vi "main.vi"() -> ()   [LabVIEW 2018]
uses:
  ctl/matrix.ctl
  <vilib>/Utility/miscctls.llb/LVRectTypeDef.ctl
  <vilib>/Utility/error.llb/DialogType.ctl
panel:
  in  "选择模式":enum16{"模式一", "模式二"}(ring)
  in  "状态刷新":bool=TRUE
  out "系统时间":timestamp format="%<%.0X\n%x>T"
  in  "setting":T1
  in  "记录数据":i32=1 min=1 step=1
  out "系统状态":string
  out "运行中":bool
  in  "初始化":T1
  in  "停止":T1
  in  "开始测试":T1
  in  "停止变量":bool=TRUE
  out "第二行":T2
  out "第一行":T2
  # "气罐压力信号数据采集系统"
  # "轮"
  # "X1\n丨"
  # "X5\n丨"
  # "X10\n 丨"
  # "X15\n 丨"
  # "X20\n 丨"
  # "X25\n 丨"
  # "X30\n 丨"
  # "X35\n 丨"
  # "X40\n 丨"
  # "X45\n 丨"
  # "X50\n 丨"
  # "X55\n 丨"
  # "X60\n 丨"
  # "X64\n 丨"
  # "Y1一"
  # "Y2一"
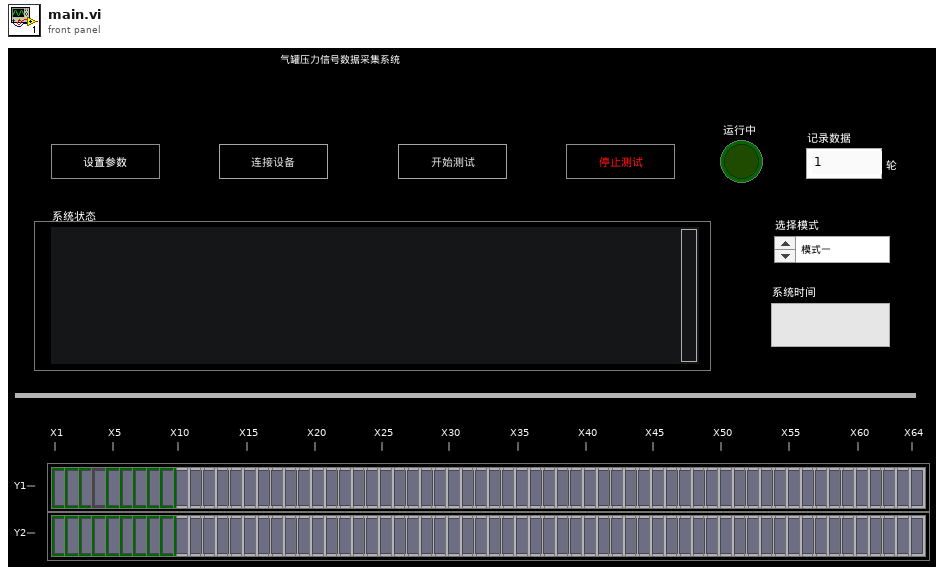
[diagram p1: front panel]
types:
  T1 = typedef "空白按钮.ctl" = bool
  T2 = typedef "matrix.ctl" = cluster{"布尔":bool, "布尔 2":bool, "布尔 3":bool, "布尔 4":bool, "布尔 5":bool, "布尔 6":bool, "布尔 7":bool, "布尔 8":bool, "布尔 9":bool, "布尔 10":bool, "布尔 11":bool, "布尔 12":bool, "布尔 13":bool, "布尔 14":bool, "布尔 15":bool, "布尔 16":bool, "布尔 17":bool, "布尔 18":bool, "布尔 19":bool, "布尔 20":bool, "布尔 21":bool, "布尔 22":bool, "布尔 23":bool, "布尔 24":bool, "布尔 25":bool, "布尔 26":bool, "布尔 27":bool, "布尔 28":bool, "布尔 29":bool, "布尔 30":bool, "布尔 31":bool, "布尔 32":bool, "布尔 33":bool, "布尔 34":bool, "布尔 35":bool, "布尔 36":bool, "布尔 37":bool, "布尔 38":bool, "布尔 39":bool, "布尔 40":bool, "布尔 41":bool, "布尔 42":bool, "布尔 43":bool, "布尔 44":bool, "布尔 45":bool, "布尔 46":bool, "布尔 47":bool, "布尔 48":bool, "布尔 49":bool, "布尔 50":bool, "布尔 51":bool, "布尔 52":bool, "布尔 53":bool, "布尔 54":bool, "布尔 55":bool, "布尔 56":bool, "布尔 57":bool, "布尔 58":bool, "布尔 59":bool, "布尔 60":bool, "布尔 61":bool, "布尔 62":bool, "布尔 63":bool, "布尔 64":bool}
  T3 = enum16{"错误", "关闭", "系统停止", "系统运行", "系统空闲", "初始化完成", "保存参数", "手动连接", "自动连接", "初始化"}
  T4 = enum32{"Invalid", "Standard", "Closed", "Hidden", "Minimized", "Maximized"}
  T5 = enum8{"Enabled", "Disabled", "Disabled and Grayed Out"}
  T6 = typedef "DialogType.ctl" = u16
  T7 = cluster{"矩阵卡设置":cluster{"BUS":u32, "slot":u32}, "模式一设置":cluster{"M1-drive-start":u32, "M1-drive-num":u32, "M1-receive-start":u32, "M1-receive-num":u32, "M1-start-delay":u32, "M1-receive-delay":u32}, "模式二设置":cluster{"M2-drive-start":u32, "M2-receive-start":u32, "M2-receive-num":u32, "M2-start-delay":u32, "M2-receive-delay":u32}, "采集设置":cluster{"Resource Name":refnum<k15>, "Input Impedance":u32, "采集通道":i32, "Trigger Level (V)":dbl, "Coupling":u16, "Trigger Slope":i32, "Min Record Length":i32, "Min. Sample Rate":dbl, "Vertical Range (V)":dbl, "触发通道":i32}}
  T8 = typedef "LVRectTypeDef.ctl" = cluster{"Left":i16, "Top":i16, "Right":i16, "Bottom":i16}
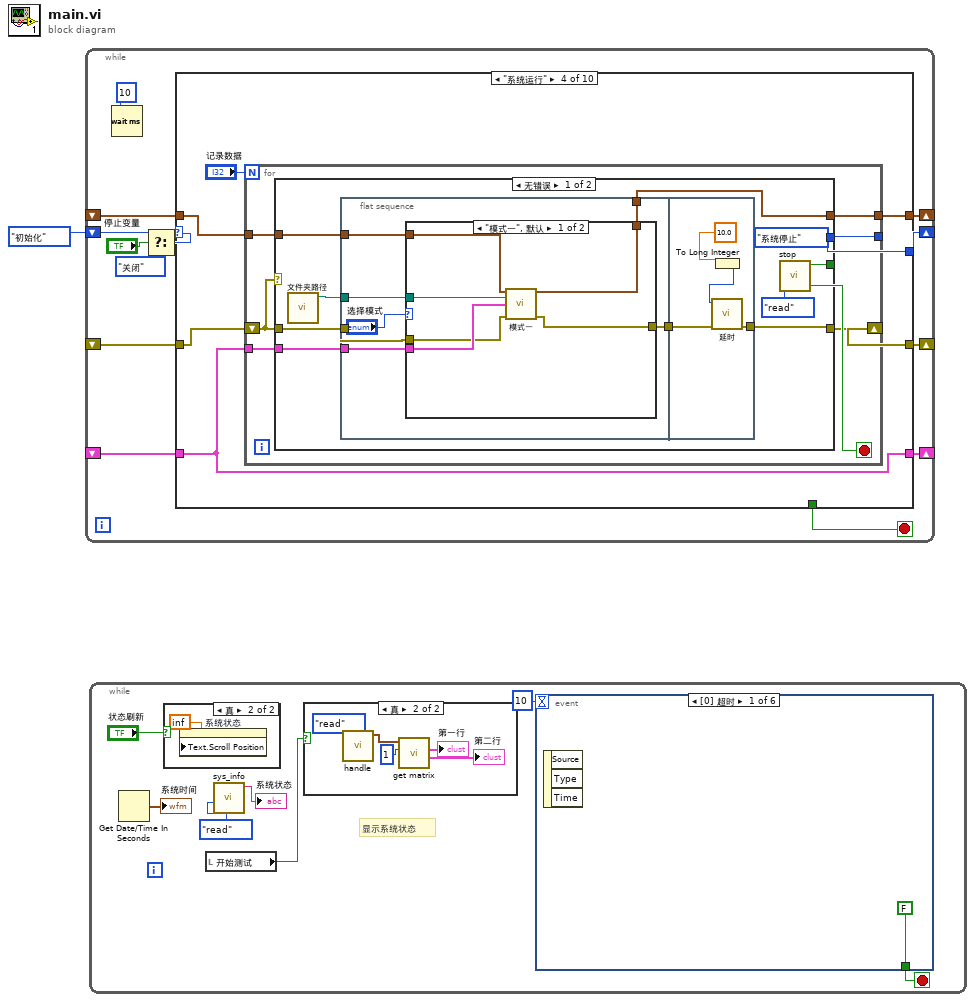
[diagram p0: block diagram]
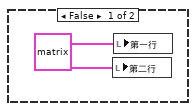
[diagram p2: hidden frame]
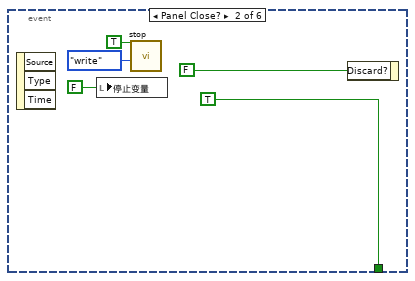
[diagram p4: hidden frame]
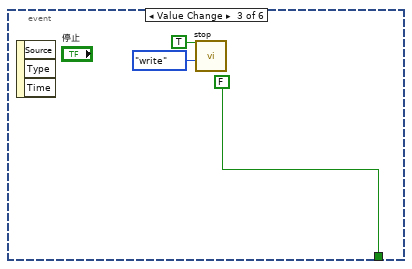
[diagram p5: hidden frame]
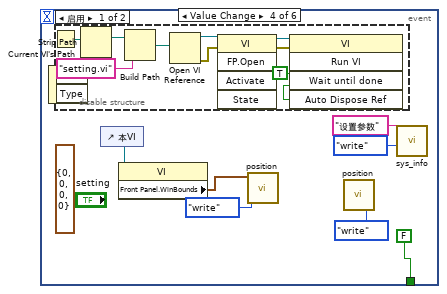
[diagram p6: hidden frame]
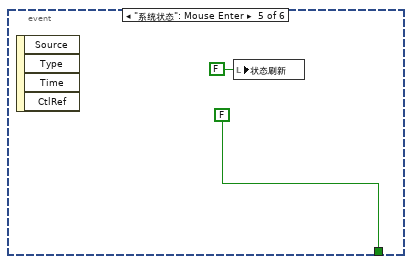
[diagram p8: hidden frame]
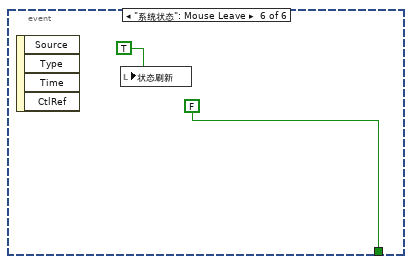
[diagram p9: hidden frame]
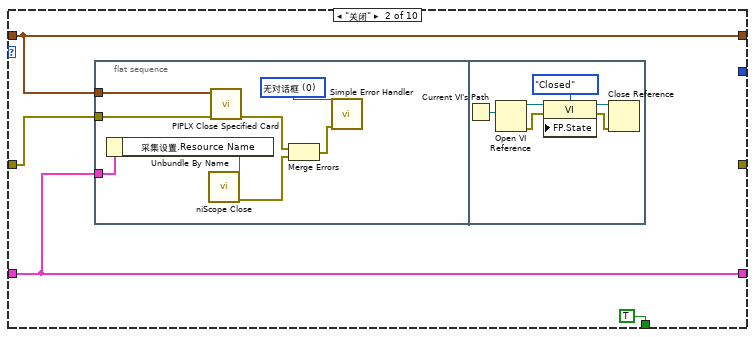
[diagram p11: hidden frame]
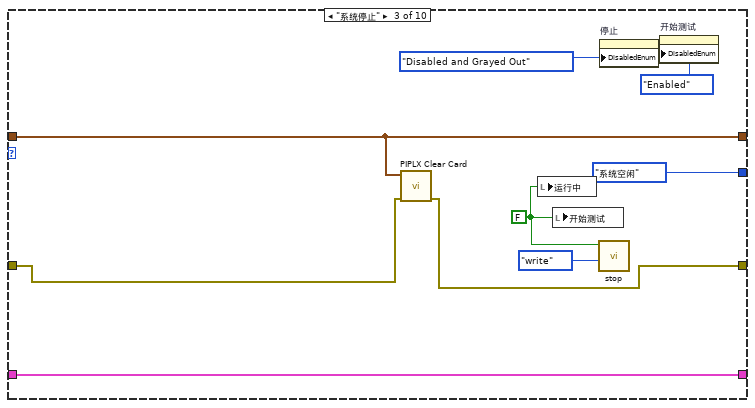
[diagram p12: hidden frame]
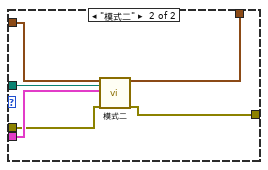
[diagram p13: hidden frame]
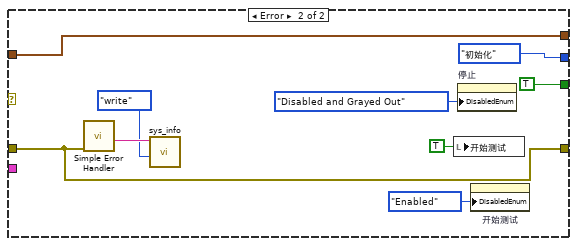
[diagram p14: hidden frame]
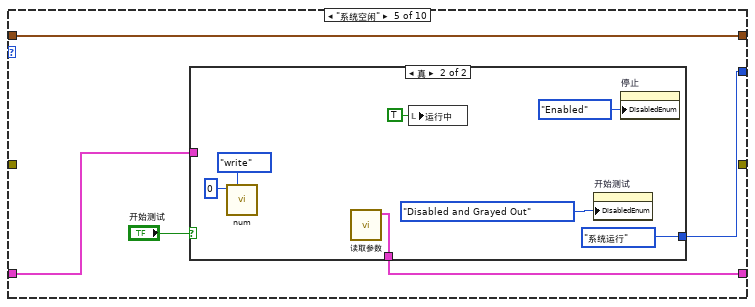
[diagram p15: hidden frame]
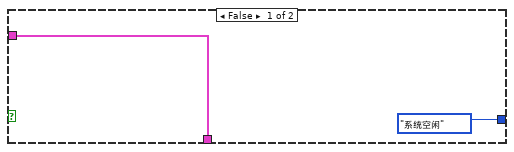
[diagram p16: hidden frame]
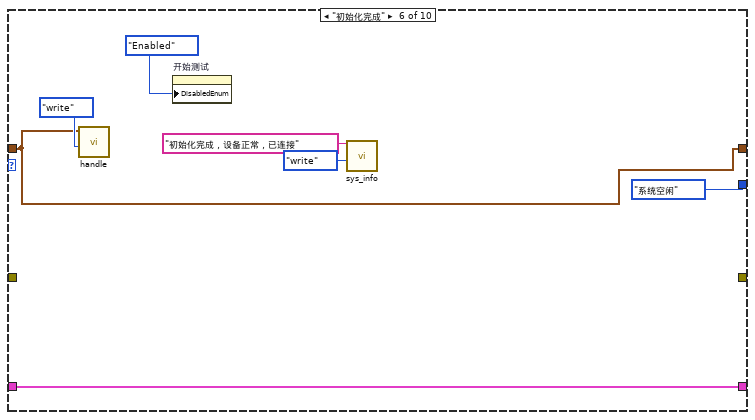
[diagram p17: hidden frame]
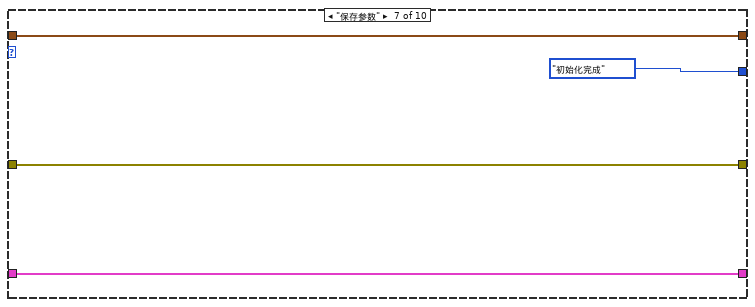
[diagram p18: hidden frame]
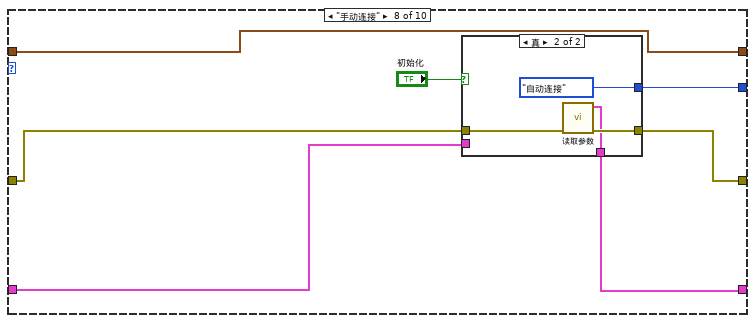
[diagram p19: hidden frame]
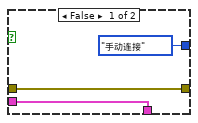
[diagram p20: hidden frame]
diagram:
  n1 = while {
    shift-right: [w14] -> _
    shift-left: T3."初始化" ("流程") -> [w12]
    shift-right: [w8] -> _
    shift-left: _ -> [w7]
    shift-right: [w5] -> _
    shift-left: _ -> [w4]
    shift-right: [w3] -> _
    shift-left: _ -> [w2]
    stop <- w6 stop-if-true
    n2 = Wait (ms)(milliseconds to wait=u32 10 ("等待时间（毫秒）")) -> ()  [unwired: 1 out]
    n3 = Select(t=w12, s="停止变量", f=T3."关闭") -> (s? t:f=w11:T3)
    n4 = case shown="\"系统运行\"" w11 {
      tunnel: [_ _ T3."系统空闲" ("流程") w50 w104 T3."系统空闲" ("流程") T3."初始化完成" ("流程") w131 w144 T3."自动连接" ("流程")] -> w14
      tunnel: [_ _ w39 w49 _ _ w122 w128 _ _] -> w8
      tunnel: w7 -> [_ w19 w40 w47 _ _ w122 w129 _ w157]
      tunnel: [_ TRUE _ _ _ _ _ _ _ _] -> w6
      tunnel: [w15 w17 w36 w45 w101 w114 w123 w130 w140 w156] -> w5
      tunnel: w4 -> [w15 w17 w36 w45 w100 w114 w123 w127 w140 _]
      tunnel: [w16 w18 w35 w44 w102 w117 w121 w125 w142 w158] -> w3
      tunnel: w2 -> [w16 w18 w35 w46 w102 w117 w121 w125 _ w158]
      frame "错误" {
      }
      frame "关闭" {
        n5 = flat-sequence {
          tunnel: w19 -> [w27]
          tunnel: w18 -> [w26]
          tunnel: w17 -> [w25]
          frame #0 {
            w28 = T6 0 items=["无对话框", "确定信息", "继续或停止信息", "确定信息＋警告", "继续/停止+警告"] ("type of dialog (OK msg:1)")
            n6 = Unbundle By Name(w25) -> ("采集设置.Resource Name"=w24:refnum<k15>)
            n7 = call <instrlib>:"niScope Close.vi"("instrument handle"=w24) -> ("error out"=w22:errorcluster)  [unwired: 14 in]
            n8 = call <instrlib>:"PIPLX Close Specified Card.vi"("error in"=w27, "Input Handle"=w26) -> ("error out"=w23:errorcluster)  [unwired: 8 in, 1 out]
            n9 = Merge Errors(w23, w22) -> (w21:errorcluster)
            n10 = call <vilib>:"Simple Error Handler.vi"("type of dialog (OK msg:1)"=w28, "error in (no error)"=w21) -> ()  [unwired: 3 in, 5 out]
          }
          frame #1 {
            n11 = Current VI's Path() -> (path=w34:path)
            n12 = Open VI Reference(vi path=w34) -> (vi reference=w33:refnum<vi>, error out=w31:errorcluster)  [unwired: 5 in]
            n13 = property class="VI"(reference=w33, error in=w31, "FP.State"=T4."Closed" ("前面板窗口:状态")) -> (reference out=w29:refnum<vi>, error out=w30:errorcluster)
            n14 = Close Reference(reference=w29, error in (no error)=w30) -> ()  [unwired: 1 out]
          }
        }
      }
      frame "系统停止" {
        w41 = FALSE ("开始按钮")
        n15 = call <instrlib>:"PIPLX Clear Card.vi"("error in"=w40, "Input Handle"=w35) -> ("error out"=w39:errorcluster)  [unwired: 8 in, 1 out]
        n16 = local write "运行中"(w41) -> ()
        n17 = local write "开始测试"(w41) -> ()
        n18 = call "stop.vi"("枚举"=enum16{"write", "read"}."write", "停止"=w41) -> ()  [unwired: 9 in, 1 out]
        n19 = property on="停止" class="Bool"("DisabledEnum"=T5."Disabled and Grayed Out" ("禁用")) -> ()  [unwired: 2 in, 2 out]
        n20 = property on="开始测试" class="Bool (严格)"("DisabledEnum"=T5."Enabled" ("禁用")) -> ()  [unwired: 2 in, 2 out]
      }
      frame "系统运行" {
        n21 = for {
          N: "记录数据" -> [_]
          tunnel: [w57] -> w50
          shift-right: [w55] -> w49
          shift-left: w47 -> [w54]
          tunnel: w46 -> [w53]
          tunnel: w45 -> [w52]
          tunnel: [w51] -> w44
          stop <- w56 stop-if-true
          n22 = case shown="无错误" w54 {
            tunnel: [w67 TRUE ("停止")] -> w56
            tunnel: [T3."系统停止" ("流程") T3."初始化" ("流程")] -> w57
            tunnel: [w60 w92] -> w55
            tunnel: w54 -> [w62 w92]
            tunnel: w53 -> [w64 w91]
            tunnel: w52 -> [w63 _]
            tunnel: [w59 w91] -> w51
            frame No Error {
              n23 = call "文件夹路径.vi"() -> ("appended path"=w58:path)  [unwired: 11 in]
              n24 = flat-sequence {
                tunnel: w64 -> [w73]
                tunnel: w63 -> [w72]
                tunnel: w62 -> [w71]
                tunnel: [w70] -> w61
                tunnel: [w69] -> w59
                tunnel: w58 -> [w68]
                tunnel: w61 -> [w88]
                tunnel: [w87] -> w60
                frame #0 {
                  n25 = case shown="\"模式一\", 默认" "选择模式" {
                    tunnel: w73 -> [w80 w86]
                    tunnel: w72 -> [w79 w85]
                    tunnel: w71 -> [w78 w84]
                    tunnel: [w77 w83] -> w70
                    tunnel: [w76 w82] -> w69
                    tunnel: w68 -> [w75 w81]
                    frame "模式一", Default {
                      n26 = call "模式一.vi"("Input Handle"=w80, "文件夹路径"=w75, "设置"=w79, "error in"=w78) -> ("Output Handle"=w76:cluster{"Session":u32, "Card number":u32}, "error out"=w77:errorcluster)  [unwired: 10 in]
                    }
                    frame "模式二" {
                      n27 = call "模式二.vi"("Input Handle"=w86, "文件夹路径"=w81, "设置"=w85, "error in"=w84) -> ("Output Handle"=w82:cluster{"Session":u32, "Card number":u32}, "error out"=w83:errorcluster)  [unwired: 14 in]
                    }
                  }
                }
                frame #1 {
                  n28 = To Long Integer(number=10.0 ("y")) -> (32bit integer=w90:i32)
                  n29 = call "延时.vi"("error in (no error)"=w88, "延时（百毫秒）"=w90) -> ("error out"=w87:errorcluster)  [unwired: 9 in]
                }
              }
              n30 = call "stop.vi"("枚举"=enum16{"write", "read"}."read") -> ("停止"=w67:bool)  [unwired: 10 in]
            }
            frame Error {
              n31 = call <vilib>:"Simple Error Handler.vi"("error in (no error)"=w92) -> ("source out"=w94:string)  [unwired: 4 in, 4 out]
              n32 = call "sys_info.vi"("枚举"=enum16{"write", "read"}."write", "sys_info"=w94) -> ()  [unwired: 9 in, 1 out]
              n33 = local write "开始测试"(T1 TRUE ("开始测试")) -> ()
              n34 = property on="停止" class="Bool"("DisabledEnum"=T5."Disabled and Grayed Out" ("禁用")) -> ()  [unwired: 2 in, 2 out]
              n35 = property on="开始测试" class="Bool (严格)"("DisabledEnum"=T5."Enabled" ("禁用")) -> ()  [unwired: 2 in, 2 out]
            }
          }
        }
      }
      frame "系统空闲" {
        n36 = case shown="真" "开始测试" {
          tunnel: [T3."系统空闲" ("流程") T3."系统运行" ("流程")] -> w104
          tunnel: [w105 w107] -> w101
          tunnel: w100 -> [w105 _]
          frame False {
          }
          frame True {
            n37 = call "num.vi"("枚举"=enum16{"write", "read"}."write", "num"=0) -> ()  [unwired: 9 in, 1 out]
            n38 = call "读取参数.vi"() -> ("设置"=w107:T7)  [unwired: 10 in, 1 out]
            n39 = local write "运行中"(TRUE ("运行中")) -> ()
            n40 = property on="开始测试" class="Bool (严格)"("DisabledEnum"=T5."Disabled and Grayed Out" ("禁用")) -> ()  [unwired: 2 in, 2 out]
            n41 = property on="停止" class="Bool"("DisabledEnum"=T5."Enabled" ("禁用")) -> ()  [unwired: 2 in, 2 out]
          }
        }
      }
      frame "初始化完成" {
        n42 = call "handle.vi"("枚举"=enum16{"write", "read"}."write", "In Handle"=w117) -> ()  [unwired: 9 in, 1 out]
        n43 = property on="开始测试" class="Bool (严格)"("DisabledEnum"=T5."Enabled" ("禁用")) -> ()  [unwired: 2 in, 2 out]
        n44 = call "sys_info.vi"("枚举"=enum16{"write", "read"}."write", "sys_info"="初始化完成，设备正常，已连接") -> ()  [unwired: 9 in, 1 out]
      }
      frame "保存参数" {
      }
      frame "手动连接" {
        n45 = case shown="真" "初始化" {
          tunnel: [T3."手动连接" ("流程") T3."自动连接" ("流程")] -> w131
          tunnel: [w132 w135] -> w130
          tunnel: w129 -> [w133 w137]
          tunnel: [w133 w136] -> w128
          tunnel: w127 -> [w132 _]
          frame False {
          }
          frame True {
            n46 = call "读取参数.vi"("error in (no error)"=w137) -> ("error out"=w136:errorcluster, "设置"=w135:T7)  [unwired: 9 in]
          }
        }
      }
      frame "自动连接" {
        n47 = call "conect and open A.vi"("设置"=w140, "Card ID"="40-533B-032") -> ("Output Handle"=w142:cluster{"Session":u32, "Card number":u32}, "find?"=w143:bool, "error out"=w141:errorcluster)  [unwired: 3 in]
        n48 = Or(x=w143, y=w141) -> (x .or. y?=w145:bool)
        n49 = case shown="假" w145 {
          tunnel: [T3."初始化完成" ("流程") T3."手动连接" ("流程")] -> w144
          tunnel: w141 -> [_ w152]
          frame False {
            n50 = property on="初始化" class="Bool"("DisabledEnum"=T5."Disabled and Grayed Out" ("禁用")) -> ()  [unwired: 2 in, 2 out]
            n51 = call "sys_info.vi"("枚举"=enum16{"write", "read"}."write", "sys_info"="初始化完成，设备正常，已连接") -> ()  [unwired: 9 in, 1 out]
          }
          frame True {
            w151 = T6 0 items=["无对话框", "确定信息", "继续或停止信息", "确定信息＋警告", "继续/停止+警告"] ("type of dialog (OK msg:1)")
            n52 = call <vilib>:"Simple Error Handler.vi"("type of dialog (OK msg:1)"=w151, "error in (no error)"=w152) -> ("source out"=w150:string)  [unwired: 3 in, 4 out]
            n53 = call "sys_info.vi"("枚举"=enum16{"write", "read"}."write", "sys_info"=w150) -> ()  [unwired: 9 in, 1 out]
          }
        }
      }
      frame "初始化", Default {
        w162 = T5."Disabled and Grayed Out" ("禁用")
        n54 = property on="初始化" class="Bool"("DisabledEnum"=T5."Enabled" ("禁用")) -> ()  [unwired: 2 in, 2 out]
        n55 = property on="开始测试" class="Bool (严格)"("DisabledEnum"=w162) -> ()  [unwired: 2 in, 2 out]
        n56 = property on="停止" class="Bool"("DisabledEnum"=w162) -> ()  [unwired: 2 in, 2 out]
        n57 = property on="系统状态" class="Str"("Visible"=TRUE ("可见")) -> ()  [unwired: 2 in, 2 out]
        n58 = call "sys_info.vi"("枚举"=enum16{"write", "read"}."write", "sys_info"="系统初始化...") -> ()  [unwired: 9 in, 1 out]
        n59 = disable-structure shown="禁用" {
          disable-tunnel: w157 -> [w167 _]
          frame Disabled {
            # "强制调整面板大小"
            n60 = control-ref of="本VI"() -> (w174:refnum<vi>)
            n61 = property class="VI"(reference=w174, error in=w167) -> (reference out=w171:refnum<vi>, error out=w170:errorcluster, "Front Panel.WinBounds"=w173:T8)
            n62 = call "调整窗口大小.vi"("前面板窗口:前面板边界"=w173, "x"=i16 1024, "y"=i16 591) -> ("前面板边界"=w172:T8)  [unwired: 7 in]
            n63 = property class="VI"(reference=w171, error in=w170, "Front Panel.WinBounds"=w172) -> ()  [unwired: 2 out]
          }
          frame Enabled {
          }
        }
        n64 = property on="系统状态" class="Str"("Text.TextColor"=u32 16448250 ("颜色盒")) -> ()  [unwired: 2 in, 2 out]
        n65 = property on="子面板" class="SubPnl"("Visible"=FALSE ("可见")) -> ()  [unwired: 2 in, 2 out]
        n66 = call "读取参数.vi"() -> ("设置"=w156:T7)  [unwired: 10 in, 1 out]
        "运行中" <- FALSE ("运行中")
      }
    }
  }
  n67 = while {
    stop <- w180 stop-if-true
    # "显示系统状态"
    n68 = Get Date/Time In Seconds() -> (seconds since 1Jan1904=→"系统时间":timestamp)
    n69 = case shown="真" "状态刷新" {
      frame False {
      }
      frame True {
        n70 = property on="系统状态" class="Str"("Text.Scroll Position"=inf) -> ()  [unwired: 2 in, 2 out]
      }
    }
    n71 = local read "开始测试"() -> (w175:T1)
    n72 = call "sys_info.vi"("枚举"=enum16{"write", "read"}."read") -> ("sys_info"=→"系统状态":string)  [unwired: 10 in]
    n73 = case shown="真" w175 {
      frame False {
        w182 = T2 {"布尔"=FALSE, "布尔 2"=FALSE, "布尔 3"=FALSE, "布尔 4"=FALSE, "布尔 5"=FALSE, "布尔 6"=FALSE, "布尔 7"=FALSE, "布尔 8"=FALSE, "布尔 9"=FALSE, "布尔 10"=FALSE, "布尔 11"=FALSE, "布尔 12"=FALSE, "布尔 13"=FALSE, "布尔 14"=FALSE, "布尔 15"=FALSE, "布尔 16"=FALSE, "布尔 17"=FALSE, "布尔 18"=FALSE, "布尔 19"=FALSE, "布尔 20"=FALSE, "布尔 21"=FALSE, "布尔 22"=FALSE, "布尔 23"=FALSE, "布尔 24"=FALSE, "布尔 25"=FALSE, "布尔 26"=FALSE, "布尔 27"=FALSE, "布尔 28"=FALSE, "布尔 29"=FALSE, "布尔 30"=FALSE, "布尔 31"=FALSE, "布尔 32"=FALSE, "布尔 33"=FALSE, "布尔 34"=FALSE, "布尔 35"=FALSE, "布尔 36"=FALSE, "布尔 37"=FALSE, "布尔 38"=FALSE, "布尔 39"=FALSE, "布尔 40"=FALSE, "布尔 41"=FALSE, "布尔 42"=FALSE, "布尔 43"=FALSE, "布尔 44"=FALSE, "布尔 45"=FALSE, "布尔 46"=FALSE, "布尔 47"=FALSE, "布尔 48"=FALSE, "布尔 49"=FALSE, "布尔 50"=FALSE, "布尔 51"=FALSE, "布尔 52"=FALSE, "布尔 53"=FALSE, "布尔 54"=FALSE, "布尔 55"=FALSE, "布尔 56"=FALSE, "布尔 57"=FALSE, "布尔 58"=FALSE, "布尔 59"=FALSE, "布尔 60"=FALSE, "布尔 61"=FALSE, "布尔 62"=FALSE, "布尔 63"=FALSE, "布尔 64"=FALSE} ("第一行")
        n74 = local write "第二行"(w182) -> ()
        n75 = local write "第一行"(w182) -> ()
      }
      frame True {
        n76 = call "handle.vi"("枚举"=enum16{"write", "read"}."read") -> ("Output Handle"=w185:cluster{"Session":u32, "Card number":u32})  [unwired: 10 in]
        n77 = call "get matrix.vi"("Output Subunit"=u32 1, "Input Handle"=w185) -> ("第二行"=→"第二行":T2, "第一行"=→"第一行":T2)  [unwired: 6 in, 2 out]
      }
    }
    n78 = event shown="[0] 超时" {
      selector: _ -> [_ _ _ _ _ _]
      dyn-events: _ -> [_ _ _ _ _ _]
      timeout: 10 -> [_ _ _ _ _ _]
      tunnel: [FALSE TRUE FALSE FALSE FALSE FALSE] -> w180
      event Timeout {
        n79 = event-data() -> ()  [unwired: 1 in, 3 out]
      }
      event Panel Close? {
        n80 = event-data() -> ()  [unwired: 1 in, 3 out]
        n81 = local write "停止变量"(FALSE ("布尔")) -> ()
        n82 = call "stop.vi"("枚举"=enum16{"write", "read"}."write", "停止"=TRUE) -> ()  [unwired: 9 in, 1 out]
        n83 = event-data("Discard?"=FALSE ("放弃？")) -> ()  [unwired: 1 in, 1 out]
      }
      event Value Change {
        n84 = event-data() -> ()  [unwired: 1 in, 3 out]
        n85 = call "stop.vi"("枚举"=enum16{"write", "read"}."write", "停止"=TRUE) -> ()  [unwired: 9 in, 1 out]
      }
      event Value Change {
        (unwired) T8 {"Left"=0, "Top"=0, "Right"=0, "Bottom"=0} ("前面板窗口:窗口边界")
        n86 = event-data() -> ()  [unwired: 1 in, 2 out]
        n87 = disable-structure shown="启用" {
          frame Enabled {
            w205 = TRUE ("结束前等待")
            n88 = Current VI's Path() -> (path=w213:path)
            n89 = Strip Path(path=w213) -> (stripped path=w212:path)  [unwired: 1 out]
            n90 = Build Path(base path=w212, name or relative path="setting.vi" ("名称或相对路径")) -> (appended path=w210:path)
            n91 = Open VI Reference(vi path=w210) -> (vi reference=w209:refnum<vi>, error out=w208:errorcluster)  [unwired: 5 in]
            n92 = invoke class="VI" method="FP.Open"(reference=w209, error in=w208) -> (reference out=w207:refnum<vi>, error out=w206:errorcluster)  [unwired: 3 in, 3 out]
            n93 = invoke class="VI" method="Run VI"(reference=w207, error in=w206, "Wait until done"=w205, "Auto Dispose Ref"=w205) -> ()  [unwired: 1 in, 5 out]
          }
          frame Disabled {
          }
        }
        n94 = control-ref of="本VI"() -> (w200:refnum<vi>)
        n95 = property class="VI"(reference=w200) -> ("Front Panel.WinBounds"=w199:T8)  [unwired: 1 in, 2 out]
        n96 = call "position.vi"("枚举"=enum16{"write", "read"}."write", "前面板窗口:窗口边界"=w199) -> ()  [unwired: 9 in, 1 out]
        n97 = call "position.vi"("枚举"=enum16{"write", "read"}."write") -> ()  [unwired: 10 in, 1 out]
        n98 = call "sys_info.vi"("枚举"=enum16{"write", "read"}."write", "sys_info"="设置参数") -> ()  [unwired: 9 in, 1 out]
      }
      event "系统状态": Mouse Enter {
        n99 = event-data() -> ()  [unwired: 1 in, 4 out]
        n100 = local write "状态刷新"(FALSE ("状态刷新")) -> ()
      }
      event "系统状态": Mouse Leave {
        n101 = event-data() -> ()  [unwired: 1 in, 4 out]
        n102 = local write "状态刷新"(TRUE ("状态刷新")) -> ()
      }
    }
  }
